vi "removeDuplicateTimes.vi"(8 "error in (no error)":errorcluster, 11 "ScriptEventList in":refnum<class "ScriptEventList.lvclass">) -> (0 "error out":errorcluster, 2 "list":refnum<class "ScriptEventList.lvclass">, 3 "ScriptEventList out":refnum<class "ScriptEventList.lvclass">)   [LabVIEW 2009, in "Tools.lvlib" / "Scripting.lvlib" / "ScriptEventList.lvclass"]
uses:
  ScriptEventList.lvclass
  ScriptEventList.lvclass/ScriptEventList.ctl
  ScriptEvent.lvclass
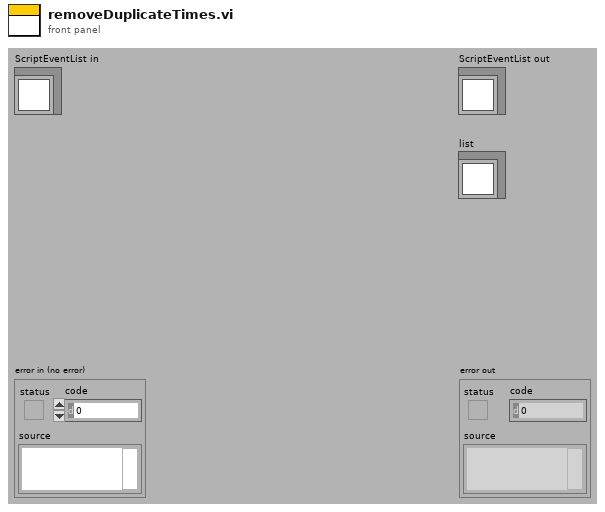
[diagram p1: front panel]
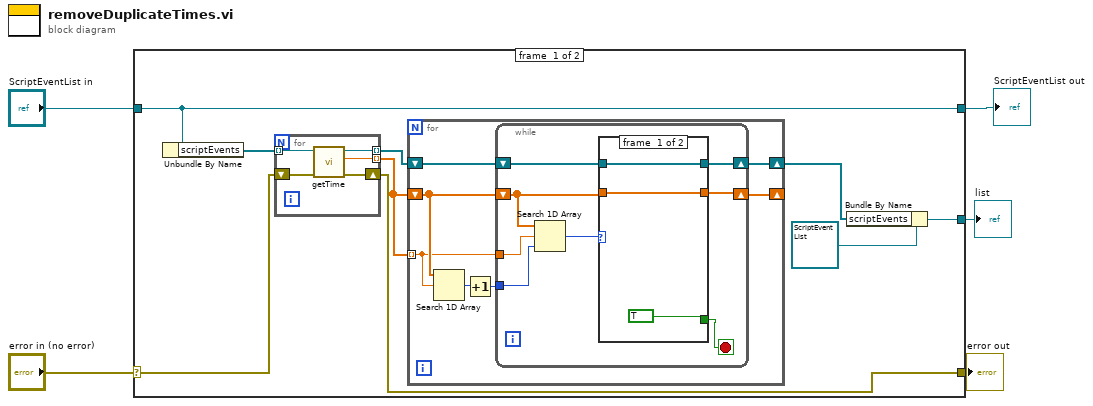
[diagram p0: block diagram]
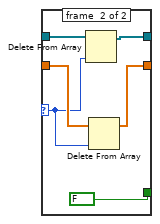
[diagram p2: hidden frame]
diagram:
  n1 = case shown="No Error" "error in (no error)" {
    selector: "error in (no error)" -> [w12 w45]
    tunnel: [w6 w45] -> w4
    tunnel: [w14 w44] -> w2
    tunnel: "ScriptEventList in" -> [w14 w44]
    tunnel: [w7 _] -> w1
    frame #0 {
      n2 = Unbundle By Name(w14) -> ("scriptEvents"=w13:refnum<class "ScriptEvent.lvclass">[])
      n3 = for {
        tunnel: w13 -> [w43] mode=indexing
        tunnel: [w41] -> w11 mode=indexing
        tunnel: [w40] -> w10 mode=indexing
        shift-right: [w39] -> w6
        shift-left: w12 -> [w42]
        n4 = call "getTime.vi"("error in (no error)"=w42, "ScriptEvent.lvclass in"=w43) -> ("error out"=w39:errorcluster, "time"=w41:dbl, "ScriptEvent.lvclass out"=w40:refnum<class "ScriptEvent.lvclass">)  [unwired: 7 in]
      }
      n5 = for {
        tunnel: w11 -> [w19] mode=indexing
        shift-right: [w21] -> _
        shift-left: w11 -> [w20]
        shift-right: [w17] -> w8
        shift-left: w10 -> [w18]
        n6 = Search 1D Array(1D array=w20, element=w19) -> (index of element=w16:i32)  [unwired: 1 in]
        n7 = Increment(x=w16) -> (x+1=w15:i32)
        n8 = while {
          tunnel: w19 -> [w29]
          shift-right: [w23] -> w21
          shift-left: w20 -> [w24]
          tunnel: w15 -> [w22]
          shift-right: [w26] -> w17
          shift-left: w18 -> [w27]
          stop <- w25 stop-if-true
          n9 = Search 1D Array(1D array=w24, element=w29, start index (0)=w22) -> (index of element=w28:i32)
          n10 = case shown="Default" w28 {
            selector: w28 -> [_ w33]
            tunnel: [TRUE FALSE] -> w25
            tunnel: w27 -> [w30 w34]
            tunnel: [w30 w35] -> w26
            tunnel: w24 -> [w31 w37]
            tunnel: [w31 w36] -> w23
            frame #0 {
            }
            frame #1 {
              n11 = Delete From Array(array=w34, index=w33) -> (array with subset deleted=w35:refnum<class "ScriptEvent.lvclass">[])  [unwired: 1 in, 1 out]
              n12 = Delete From Array(array=w37, index=w33) -> (array with subset deleted=w36:dbl[])  [unwired: 1 in, 1 out]
            }
          }
        }
      }
      n13 = Bundle By Name(cluster=refnum<class "ScriptEventList.lvclass"> refnum ("ScriptEventList in"), "scriptEvents"=w8) -> (w7:refnum<class "ScriptEventList.lvclass">)
    }
    frame #1 {
    }
  }
  "error out" <- w4
  "ScriptEventList out" <- w2
  "list" <- w1
